vi "JSON Example.vi"   [LabVIEW 2014]
uses:
  QwaveSys_Interface/QwaveSys_Interface.lvlib
  QwaveSys_ESP8266/QwaveSys_ESP8266.lvlib
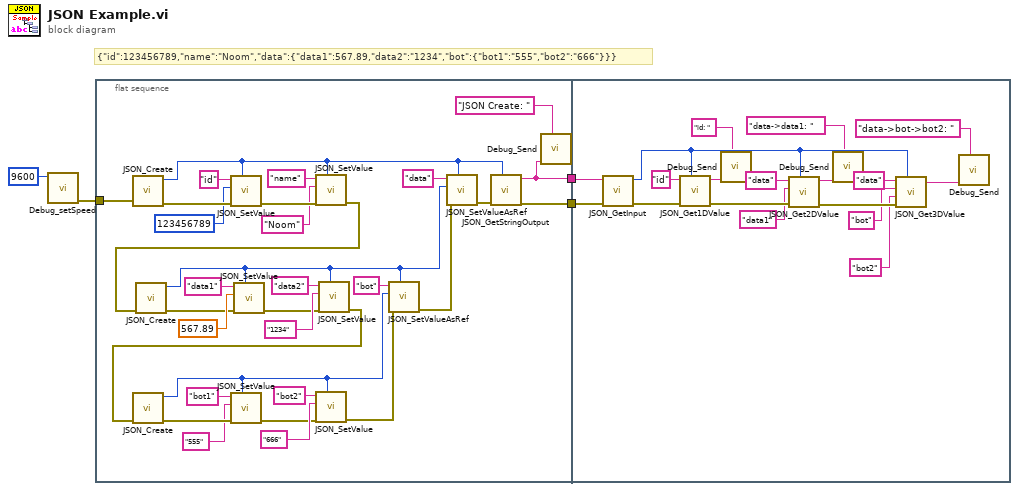
[diagram p0: block diagram]
diagram:
  # "{\"id\":123456789,\"name\":\"Noom\",\"data\":{\"data1\":567.89,\"data2\":\"1234\",\"bot\":{\"bot1\":\"555\",\"bot2\":\"666\"}}}"
  n1 = call "Debug_setSpeed.vi"("Speed"=u32 9600) -> ("error out"=w4:errorcluster)  [unwired: 10 in]
  n2 = flat-sequence {
    tunnel: w4 -> [w36]
    tunnel: [w35] -> w2
    tunnel: [w24] -> w1
    tunnel: w2 -> [w38]
    tunnel: w1 -> [w37]
    frame #0 {
      n3 = call "JSON_Create.vi"("error in (no error)"=w36) -> ("error out"=w34:errorcluster, "obj refnum"=w27:u8)  [unwired: 9 in]
      n4 = call "JSON_SetValue.vi"("json refnum"=w27, "error in (no error)"=w34, "Value"=123456789, "Key"="id") -> ("error out"=w31:errorcluster)  [unwired: 7 in]
      n5 = call "JSON_SetValue.vi"("json refnum"=w27, "error in (no error)"=w31, "Value"="Noom", "Key"="name") -> ("error out"=w8:errorcluster)  [unwired: 7 in]
      n6 = call "JSON_Create.vi"("error in (no error)"=w8) -> ("error out"=w16:errorcluster, "obj refnum"=w22:u8)  [unwired: 9 in]
      n7 = call "JSON_SetValue.vi"("json refnum"=w22, "error in (no error)"=w16, "Value"=567.89, "Key"="data1") -> ("error out"=w19:errorcluster)  [unwired: 7 in]
      n8 = call "JSON_SetValue.vi"("json refnum"=w22, "error in (no error)"=w19, "Value"="1234", "Key"="data2") -> ("error out"=w7:errorcluster)  [unwired: 7 in]
      n9 = call "JSON_Create.vi"("error in (no error)"=w7) -> ("error out"=w10:errorcluster, "obj refnum"=w23:u8)  [unwired: 9 in]
      n10 = call "JSON_SetValue.vi"("json refnum"=w23, "error in (no error)"=w10, "Value"="555", "Key"="bot1") -> ("error out"=w12:errorcluster)  [unwired: 7 in]
      n11 = call "JSON_SetValue.vi"("json refnum"=w23, "error in (no error)"=w12, "Value"="666", "Key"="bot2") -> ("error out"=w6:errorcluster)  [unwired: 7 in]
      n12 = call "JSON_SetValueAsRef.vi"("json refnum"=w22, "error in (no error)"=w6, "Value As Refnum"=w23, "Key"="bot") -> ("error out"=w5:errorcluster)  [unwired: 7 in]
      n13 = call "JSON_SetValueAsRef.vi"("json refnum"=w27, "error in (no error)"=w5, "Value As Refnum"=w22, "Key"="data") -> ("error out"=w26:errorcluster)  [unwired: 7 in]
      n14 = call "JSON_GetStringOutput.vi"("json refnum"=w27, "error in (no error)"=w26) -> ("error out"=w35:errorcluster, "json string"=w24:string)  [unwired: 8 in]
      n15 = call "Debug_Send.vi"("Name"="JSON Create: ", "DATA"=w24) -> ()  [unwired: 10 in]
    }
    frame #1 {
      n16 = call "JSON_GetInput.vi"("error in (no error)"=w38, "JSON String"=w37) -> ("error out"=w54:errorcluster, "json refnum"=w48:u8)  [unwired: 8 in]
      n17 = call "JSON_Get1DValue.vi"("json refnum"=w48, "error in (no error)"=w54, "Key"="id") -> ("error out"=w52:errorcluster, "Value"=w43:string)  [unwired: 7 in]
      n18 = call "Debug_Send.vi"("Name"="id: ", "DATA"=w43) -> ()  [unwired: 10 in]
      n19 = call "JSON_Get2DValue.vi"("json refnum"=w48, "error in (no error)"=w52, "Key2"="data1", "Key1"="data") -> ("error out"=w49:errorcluster, "Value"=w42:string)  [unwired: 6 in]
      n20 = call "Debug_Send.vi"("Name"="data->data1: ", "DATA"=w42) -> ()  [unwired: 10 in]
      n21 = call "JSON_Get3DValue.vi"("json refnum"=w48, "error in (no error)"=w49, "Key3"="bot2", "Key2"="bot", "Key1"="data") -> ("Value"=w40:string)  [unwired: 5 in, 1 out]
      n22 = call "Debug_Send.vi"("Name"="data->bot->bot2: ", "DATA"=w40) -> ()  [unwired: 10 in]
    }
  }
